vi "FSK - TESTBENCH.vi"() -> ()   [LabVIEW 2013]
uses:
  <vilib>/sound2/lvsound2.llb/Sound Data Format.ctl
  <vilib>/sound2/lvsound2.llb/Sampling Mode.ctl
  <vilib>/Analysis/3filter.llb/Zero Phase Filter (DBL).vi
  <vilib>/sound2/lvsound2.llb/Sound Output Write (DBL Single).vi
  <vilib>/Analysis/NI_AALBase.lvlib
  <vilib>/Analysis/NI_AALPro.lvlib
  <vilib>/gmath/NI_Gmath.lvlib
panel:
  out "Fm rad/s":dbl
  out "Fc rad/s":dbl
  out "Waveform Graph 2":dbl[](graph)
  in  "noise":dbl=0.2 format="%#_13g"
  out "Waveform Graph":waveform(dbl)(graph)
  in  "data length":i32=10
  out "data":string
  out "size(s)":i32
  in  "Fm MHz":dbl=15.0 format="%#_13g"
  in  "Fc MHz":dbl=140.0 format="%#_13g"
  out "time per bit":dbl
  out "total message time":dbl
  in  "Bit/s":dbl=16.0 format="%#_13g"
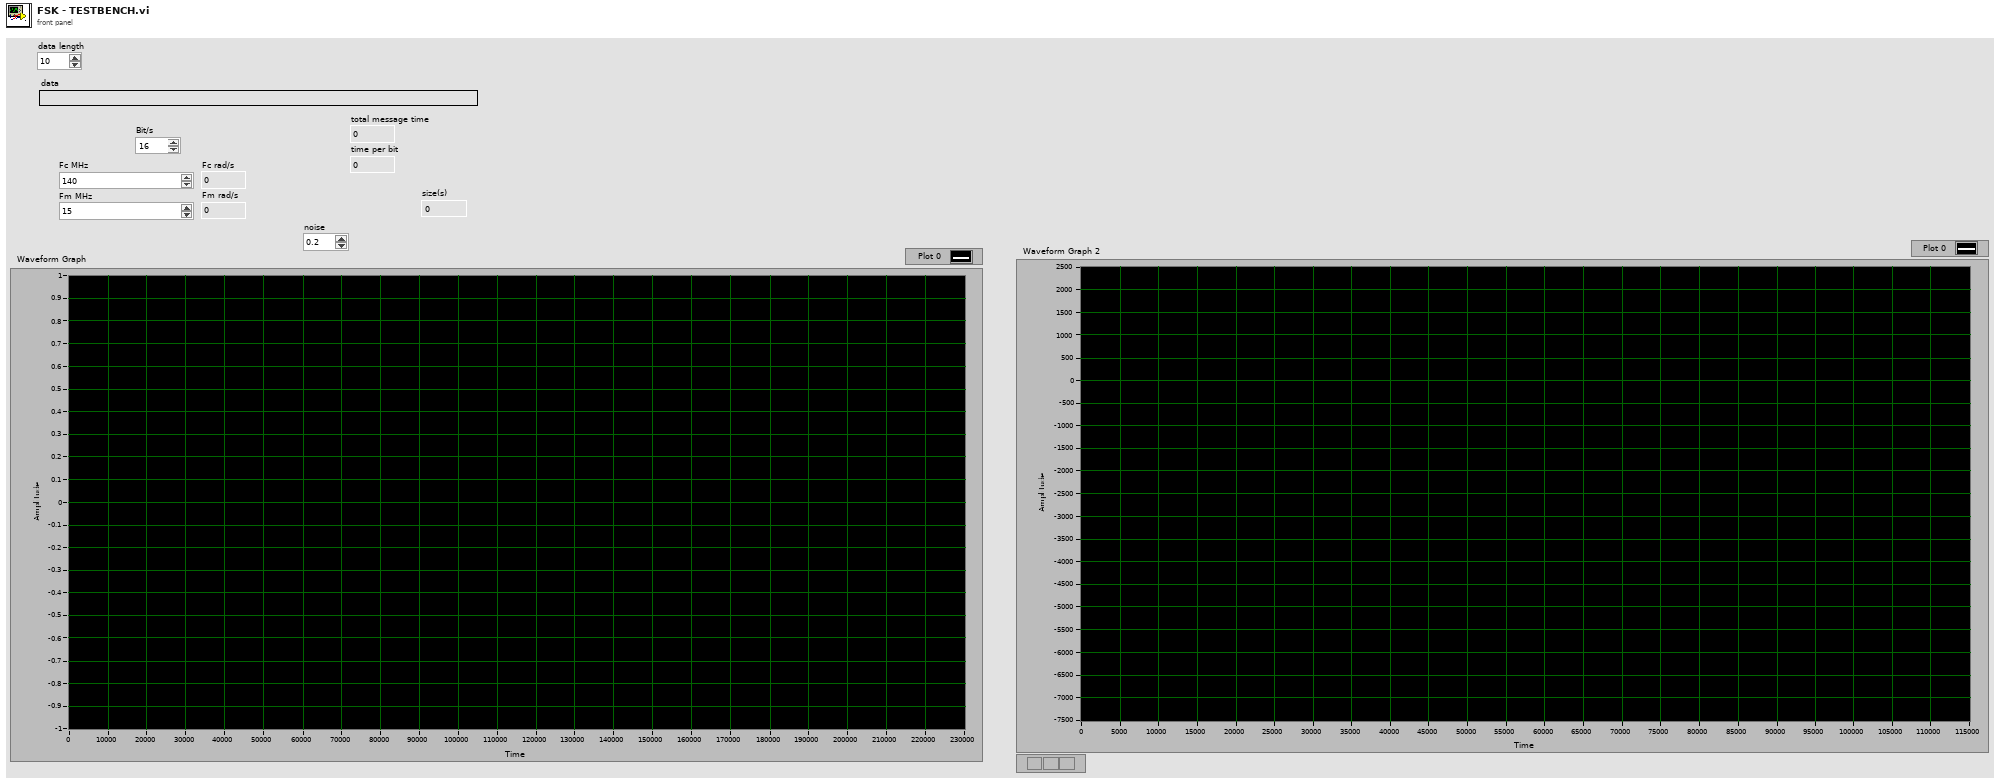
[diagram p1: front panel]
types:
  T1 = typedef "Sampling Mode.ctl" = i32
  T2 = typedef "Sound Data Format.ctl" = cluster{"sample rate (S/s)":dbl, "number of channels":i32, "bits per sample":i32}
  T3 = typedef "Sound Output Task ID.ctl" = u32
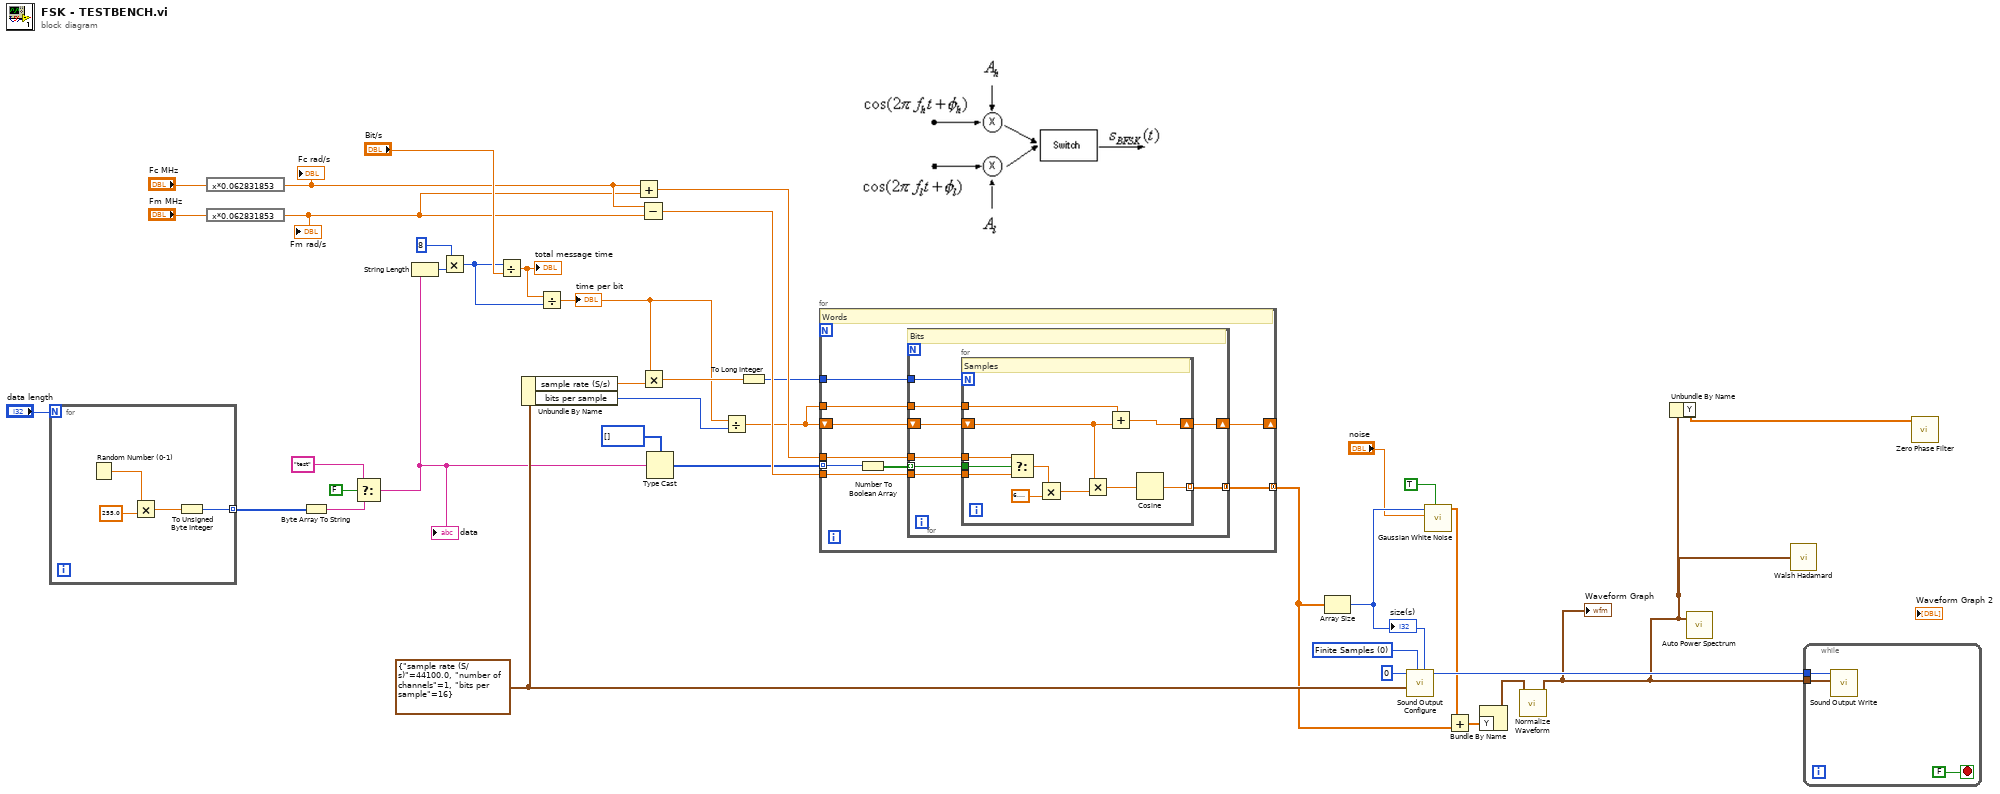
[diagram p0: block diagram]
diagram:
  w31 = T1 0 items=["Finite Samples", "Continuous Samples"] ("sample mode")
  w30 = T2 {"sample rate (S/s)"=44100.0, "number of channels"=1, "bits per sample"=16} ("sound format")
  n1 = for {
    N: "data length" -> [_]
    tunnel: [w39] -> w17 mode=indexing
    n2 = Random Number (0-1)() -> (number: 0 to 1=w42:dbl)
    n3 = Multiply(x=w42, y=255.0) -> (x*y=w40:dbl)
    n4 = To Unsigned Byte Integer(number=w40) -> (unsigned 8bit integer=w39:u8)
  }
  n5 = expression code="x*0.062831853"("Fc MHz") -> (w2:dbl)
  "Fc rad/s" <- w2
  n6 = expression code="x*0.062831853"("Fm MHz") -> (w1:dbl)
  "Fm rad/s" <- w1
  n7 = Byte Array To String(unsigned byte array=w17) -> (string=w16:string)
  n8 = Select(t="test", s=FALSE, f=w16) -> (s? t:f=w14:string)
  "data" <- w14
  n9 = String Length(string=w14) -> (length=w34:i32)
  n10 = Multiply(x=8, y=w34) -> (x*y=w33:i32)
  n11 = Divide(x=w33, y="Bit/s") -> (x/y=w35:dbl)
  "total message time" <- w35
  n12 = Unbundle By Name(w30) -> ("sample rate (S/s)"=w29:dbl, "bits per sample"=w23:i32)
  n13 = Divide(x=w35, y=w33) -> (x/y=w19:dbl)
  "time per bit" <- w19
  n14 = Add(x=w2, y=w1) -> (x+y=w27:dbl)
  n15 = Subtract(x=w2, y=w1) -> (x-y=w24:dbl)
  n16 = Multiply(x=w19, y=w29) -> (x*y=w28:dbl)
  n17 = Type Cast(type=u8[] [], x=w14) -> (*(type *) &x=w21:u8[])
  n18 = Divide(x=w19, y=w23) -> (x/y=w20:dbl)
  n19 = To Long Integer(number=w28) -> (32bit integer=w18:i32)
  n20 = for {
    tunnel: w21 -> [w51] mode=indexing
    tunnel: w18 -> [w49]
    tunnel: w27 -> [w48]
    tunnel: w24 -> [w47]
    tunnel: w20 -> [w45]
    shift-right: [w44] -> _
    shift-left: w20 -> [w46]
    tunnel: [w43] -> w3 mode=concatenating
    # "Words"
    n21 = Number To Boolean Array(number=w51) -> (Boolean array=w50:bool[])
    n22 = for {
      tunnel: w50 -> [w58] mode=indexing
      tunnel: w49 -> [w59]
      tunnel: w48 -> [w57]
      tunnel: w47 -> [w56]
      shift-right: [w53] -> w44
      shift-left: w46 -> [w55]
      tunnel: w45 -> [w54]
      tunnel: [w52] -> w43 mode=concatenating
      # "Bits"
      n23 = for {
        N: w59 -> [_]
        tunnel: w58 -> [w69]
        tunnel: w57 -> [w68]
        tunnel: w56 -> [w67]
        shift-right: [w62] -> w53
        shift-left: w55 -> [w63]
        tunnel: w54 -> [w64]
        tunnel: [w60] -> w52 mode=indexing
        # "Samples"
        n24 = Select(t=w68, s=w69, f=w67) -> (s? t:f=w66:dbl)
        n25 = Multiply(x=w66, y=6.283185307179586) -> (x*y=w65:dbl)
        n26 = Multiply(x=w63, y=w65) -> (x*y=w61:dbl)
        n27 = Add(x=w64, y=w63) -> (x+y=w62:dbl)
        n28 = Cosine(x=w61) -> (cos(x)=w60:dbl)
      }
    }
  }
  n29 = Array Size(array=w3) -> (size(s)=w11:i32)
  "size(s)" <- w11
  n30 = call <vilib>:"Sound Output Configure.vi"("number of samples/ch"=w11, "sample mode"=w31, "sound format"=w30, "device ID"=u32 0) -> ("task ID"=w22:T3)  [unwired: 6 in, 1 out]
  n31 = call <vilib>:"Gaussian White Noise.vi"("initialize?"=TRUE, "standard deviation"="noise", "samples"=w11) -> ("Gaussian noise pattern"=w8:dbl[])  [unwired: 7 in, 1 out]
  n32 = Add(x=w8, y=w3) -> (x+y=w7:dbl[])
  n33 = Bundle By Name("Y"=w7) -> (w6:waveform(dbl))  [unwired: 1 in]
  n34 = call <vilib>:"Normalize Waveform.vi"("waveform in"=w6) -> ("normalized waveform"=w5:waveform(dbl))  [unwired: 7 in, 3 out]
  "Waveform Graph" <- w5
  n35 = Unbundle By Name(w5) -> ("Y"=w4:dbl[])
  n36 = call <vilib>:"Auto Power Spectrum.vi"("Signal (V)"=w5) -> ()  [unwired: 1 in, 2 out]
  n37 = call <vilib>:"Walsh Hadamard.vi"("X"=w5) -> ()  [unwired: 2 out]
  n38 = while {
    tunnel: w22 -> [w71]
    tunnel: w5 -> [w73]
    stop <- FALSE stop-if-true
    n39 = call-poly <vilib>:"Sound Output Write.vi"("data"=w73, "task ID"=w71) -> ()  [unwired: 8 in, 2 out]
  }
  n40 = call-poly <vilib>:"Zero Phase Filter.vi"("X"=w4) -> ()  [unwired: 9 in, 2 out]
